vi "niSync Initialize Advanced.vi"(0 "resource name":refnum<k15>, 5 "remote target":string, 7 "reset device":bool caption="reset device (False)", 9 "id query":bool caption="id query (True)", 11 "error in":errorcluster) -> (4 "instrument handle out":refnum<k15>, 15 "error out":errorcluster)   [LabVIEW 2024, in "NI Synchronization System Explorer.lvlib"]
uses:
  NI Synchronization System Explorer.lvlib
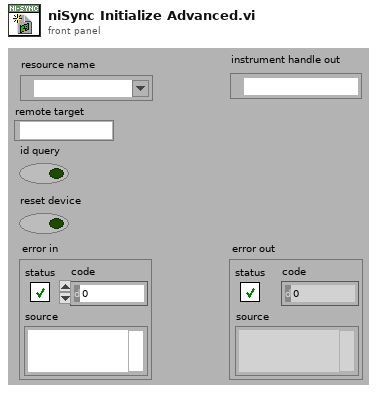
[diagram p1: front panel]
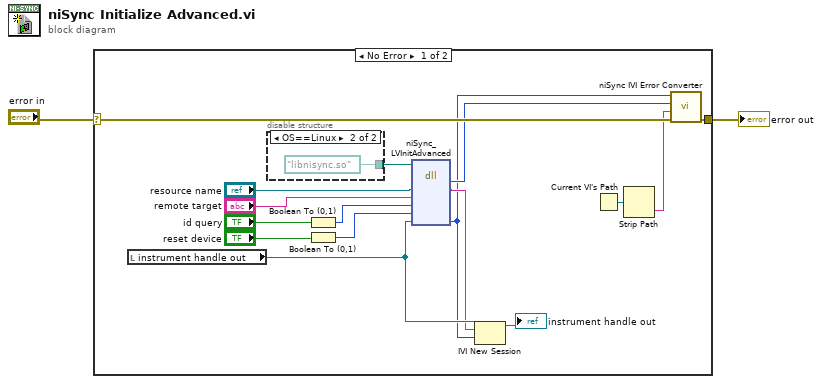
[diagram p0: block diagram]
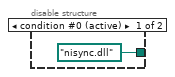
[diagram p2: hidden frame]
diagram:
  n1 = case shown="No Error" "error in" {
    selector: "error in" -> [w14 w21]
    tunnel: [w15 w21] -> w1
    frame No Error {
      n2 = local read "instrument handle out"() -> (w7:refnum<k15>)
      n3 = disable-structure shown="OS==Linux" {
        disable-tunnel: [path "nisync.dll" ("path in") path "libnisync.so" ("path in")] -> w3
        frame condition #0 (active) {
        }
        frame condition #1 {
        }
      }
      n4 = Boolean To (0,1)(Boolean="id query") -> (0, 1=w9:i16)
      n5 = Boolean To (0,1)(Boolean="reset device") -> (0, 1=w8:i16)
      n6 = dll-call lib="niSync.dll" fn="niSync_LVInitAdvanced"(path in=w3, "resource name"="resource name", "remote target"="remote target", "id query"=w9, "reset device"=w8, "instrument handle"=w7) -> ("return type"=w5:i32, "resource name"=w6:string, "instrument handle"=w4:u32)  [unwired: 5 in, 2 out]
      n7 = IVI New Session(9:w4, 10:w6, 11:w7) -> (3:→"instrument handle out":refnum<k15>)
      n8 = Current VI's Path() -> (path=w13:path)
      n9 = Strip Path(path=w13) -> (name=w12:string)  [unwired: 1 out]
      n10 = call <instrlib>:"niSync IVI Error Converter.vi"("error in (no error)"=w14, "name of VI (\"\")"=w12, "IVI error code (0)"=w5, "instrument handle (None)"=w4) -> ("error out"=w15:errorcluster)  [unwired: 6 in, 1 out]
    }
    frame Error {
    }
  }
  "error out" <- w1
